vi "Write Device.vi"(8 "error in (no error)":errorcluster, 10 "Device":string, 11 "Configuration in":refnum<class "Configuration.lvclass">) -> (0 "error out":errorcluster, 3 "Configuration out":refnum<class "Configuration.lvclass">)   [LabVIEW 2023, in "Configuration.lvlib" / "Configuration.lvclass"]
doc: "Writing a device handle to this method results in a refresh of the config.ini file and the signal list which then downselects the signal list data for the specific device."
uses:
  Library/Configuration.lvclass
  Library/Configuration.lvclass/Configuration.ctl
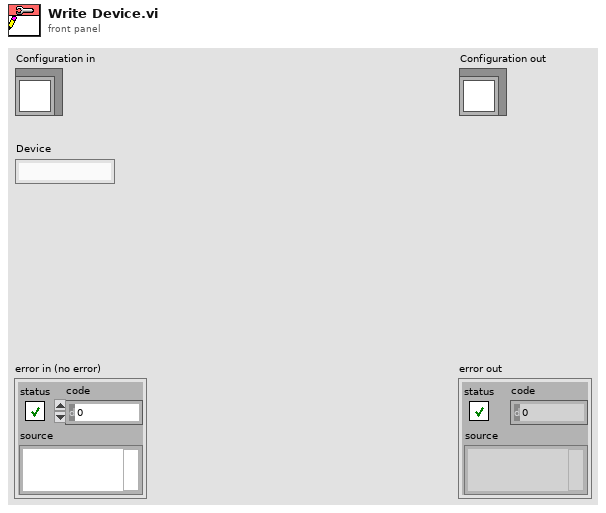
[diagram p1: front panel]
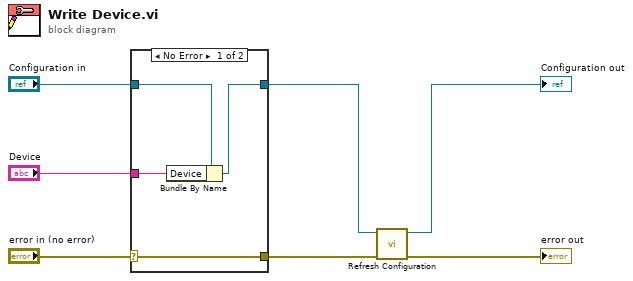
[diagram p0: block diagram]
diagram:
  n1 = case shown="No Error" "error in (no error)" {
    selector: "error in (no error)" -> [w11 w12]
    tunnel: [w11 w12] -> w4
    tunnel: [w9 w13] -> w2
    tunnel: "Configuration in" -> [w10 w13]
    tunnel: "Device" -> [w8 _]
    frame No Error {
      n2 = Bundle By Name(cluster=w10, "Device"=w8) -> (w9:refnum<class "Configuration.lvclass">)
    }
    frame Error {
    }
  }
  n3 = call "Refresh Configuration.vi"("error in (no error)"=w4, "Configuration in"=w2) -> ("error out"=→"error out":errorcluster, "Configuration out"=→"Configuration out":refnum<class "Configuration.lvclass">)  [unwired: 8 in]
